vi "Target Vision Processing.vi"(3 "Particle Measurements (COG)":dbl[][](array[numeric]) format="%.2f", 5 "Rectangles (Shape Detection 1)":T1(array[cluster]) {"Corners"."Y" format="%.2f"; "Corners"."X" format="%.2f"}) -> (0 "Chosen X":dbl, 1 "Chosen Distance":dbl, 2 "High Y":dbl)   [LabVIEW 2012]
panel:
  in  "Numeric":dbl
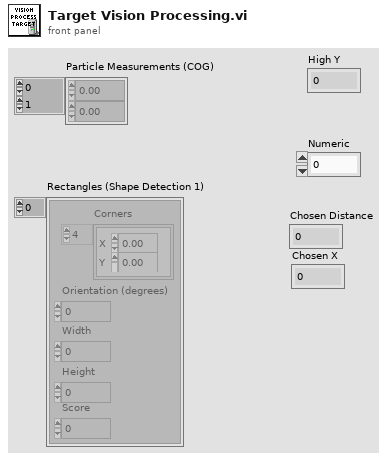
[diagram p1: front panel]
types:
  T1 = cluster{"Corners":cluster{"X":sgl, "Y":sgl}[], "Orientation (degrees)":dbl, "Width":dbl, "Height":dbl, "Score":dbl}[]
  T2 = cluster{"Rectangles (Shape Detection 1)[0]":cluster{"Corners":cluster{"X":sgl, "Y":sgl}[], "Orientation (degrees)":dbl, "Width":dbl, "Height":dbl, "Score":dbl}, "Rectangles (Shape Detection 1)[1]":cluster{"Corners":cluster{"X":sgl, "Y":sgl}[], "Orientation (degrees)":dbl, "Width":dbl, "Height":dbl, "Score":dbl}, "Rectangles (Shape Detection 1)[2]":cluster{"Corners":cluster{"X":sgl, "Y":sgl}[], "Orientation (degrees)":dbl, "Width":dbl, "Height":dbl, "Score":dbl}, "Rectangles (Shape Detection 1)[3]":cluster{"Corners":cluster{"X":sgl, "Y":sgl}[], "Orientation (degrees)":dbl, "Width":dbl, "Height":dbl, "Score":dbl}, "Rectangles (Shape Detection 1)[4]":cluster{"Corners":cluster{"X":sgl, "Y":sgl}[], "Orientation (degrees)":dbl, "Width":dbl, "Height":dbl, "Score":dbl}, "Rectangles (Shape Detection 1)[5]":cluster{"Corners":cluster{"X":sgl, "Y":sgl}[], "Orientation (degrees)":dbl, "Width":dbl, "Height":dbl, "Score":dbl}, "Rectangles (Shape Detection 1)[6]":cluster{"Corners":cluster{"X":sgl, "Y":sgl}[], "Orientation (degrees)":dbl, "Width":dbl, "Height":dbl, "Score":dbl}, "Rectangles (Shape Detection 1)[7]":cluster{"Corners":cluster{"X":sgl, "Y":sgl}[], "Orientation (degrees)":dbl, "Width":dbl, "Height":dbl, "Score":dbl}, "Rectangles (Shape Detection 1)[8]":cluster{"Corners":cluster{"X":sgl, "Y":sgl}[], "Orientation (degrees)":dbl, "Width":dbl, "Height":dbl, "Score":dbl}}
  T3 = cluster{"Corners":cluster{"X":sgl, "Y":sgl}[], "Orientation (degrees)":dbl, "Width":dbl, "Height":dbl, "Score":dbl}
  T4 = cluster{"Corners[0]":cluster{"X":sgl, "Y":sgl}, "Corners[1]":cluster{"X":sgl, "Y":sgl}, "Corners[2]":cluster{"X":sgl, "Y":sgl}, "Corners[3]":cluster{"X":sgl, "Y":sgl}, "Corners[4]":cluster{"X":sgl, "Y":sgl}, "Corners[5]":cluster{"X":sgl, "Y":sgl}, "Corners[6]":cluster{"X":sgl, "Y":sgl}, "Corners[7]":cluster{"X":sgl, "Y":sgl}, "Corners[8]":cluster{"X":sgl, "Y":sgl}}
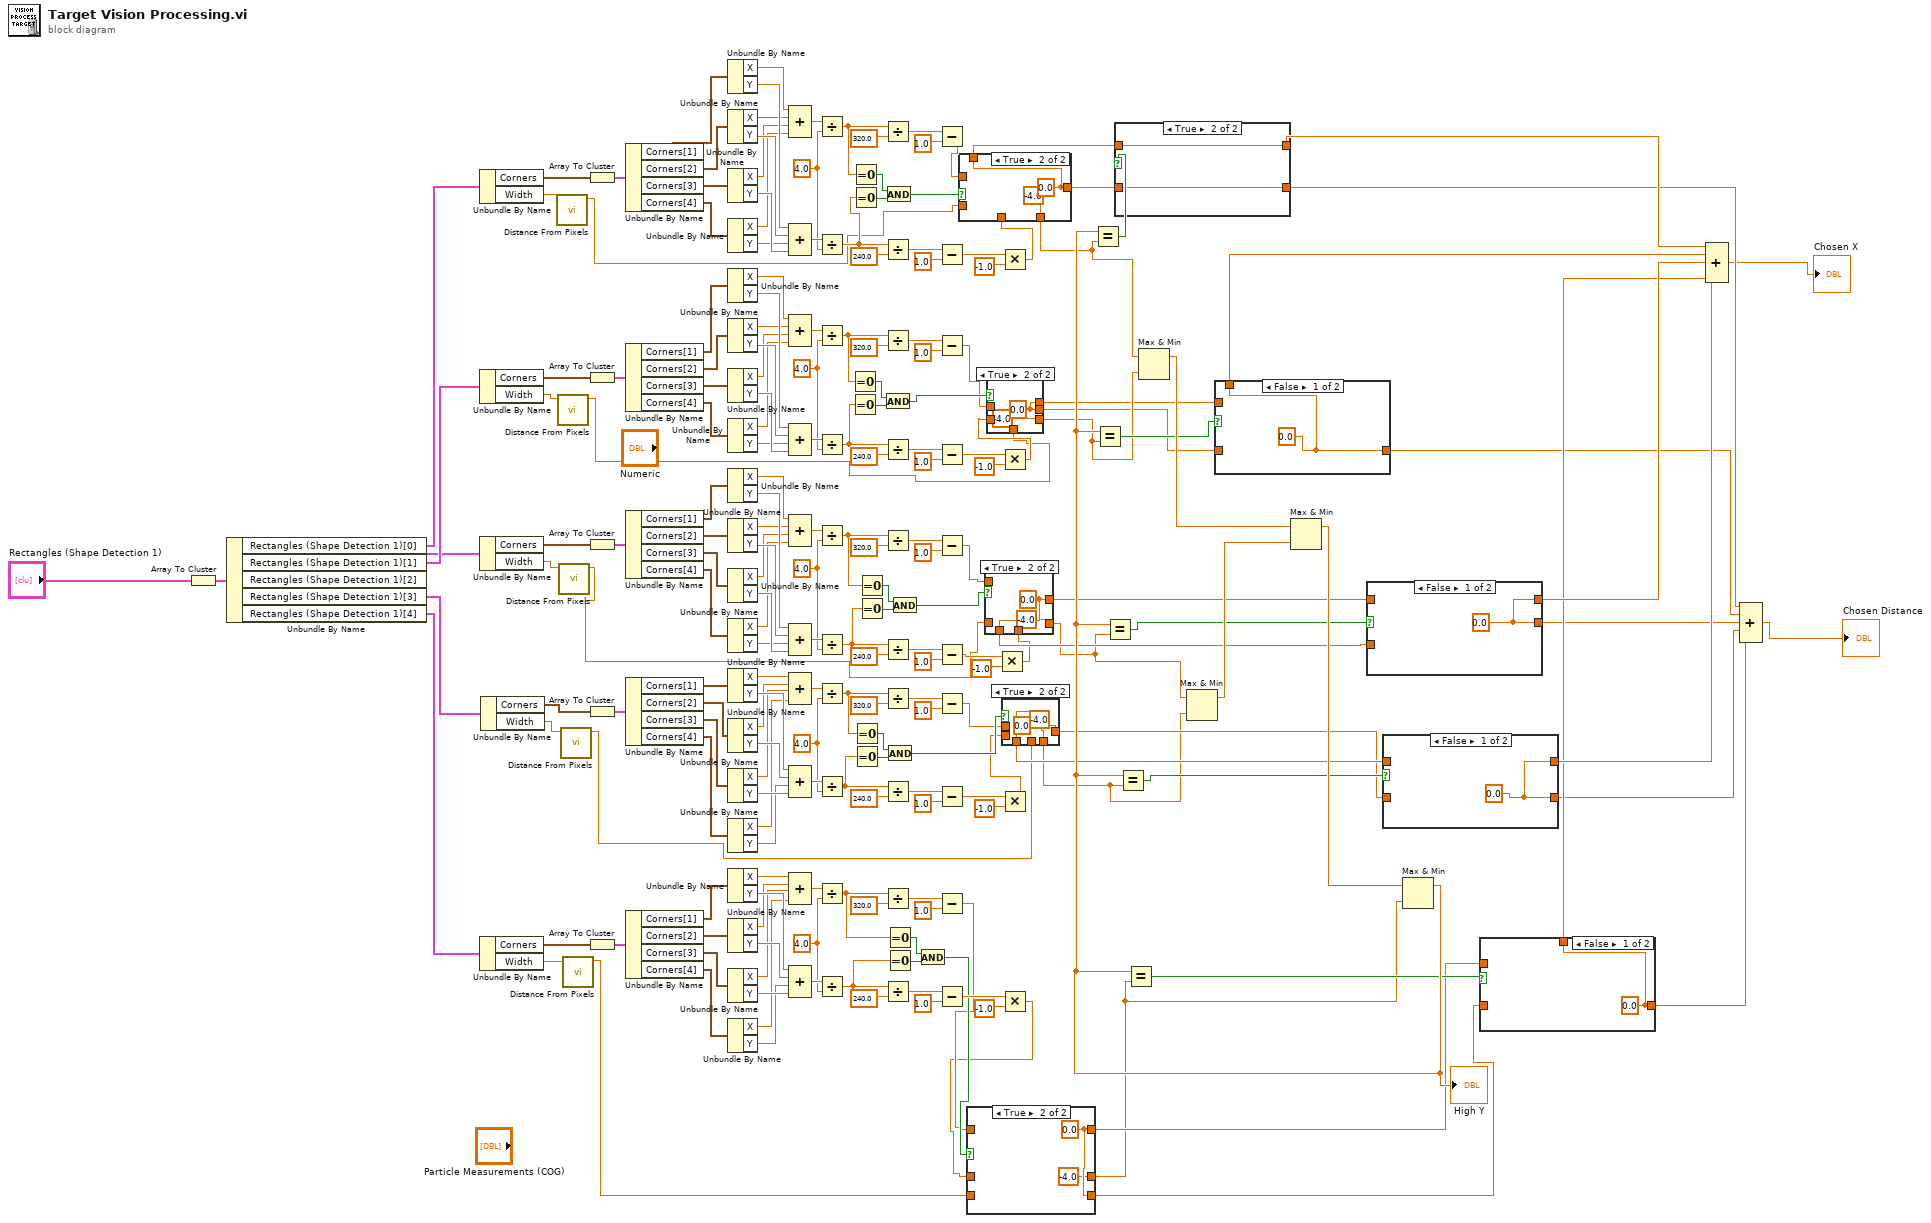
[diagram p0: block diagram]
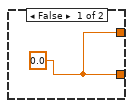
[diagram p11: hidden frame]
diagram:
  w92 = sgl 4.0 ("y")
  w117 = sgl 4.0 ("y")
  w141 = sgl 4.0 ("y")
  w166 = sgl 4.0 ("y")
  w190 = sgl 4.0 ("y")
  n1 = Array To Cluster(array="Rectangles (Shape Detection 1)") -> (cluster=w212:T2)
  n2 = Unbundle By Name(w212) -> ("Rectangles (Shape Detection 1)[0]"=w211:T3, "Rectangles (Shape Detection 1)[1]"=w210:T3, "Rectangles (Shape Detection 1)[2]"=w209:T3, "Rectangles (Shape Detection 1)[3]"=w208:T3, "Rectangles (Shape Detection 1)[4]"=w207:T3)
  n3 = Unbundle By Name(w211) -> ("Corners"=w206:cluster{"X":sgl, "Y":sgl}[], "Width"=w81:dbl)
  n4 = Unbundle By Name(w210) -> ("Corners"=w157:cluster{"X":sgl, "Y":sgl}[], "Width"=w77:dbl)
  n5 = Unbundle By Name(w209) -> ("Corners"=w133:cluster{"X":sgl, "Y":sgl}[], "Width"=w78:dbl)
  n6 = Unbundle By Name(w207) -> ("Corners"=w83:cluster{"X":sgl, "Y":sgl}[], "Width"=w80:dbl)
  n7 = Unbundle By Name(w208) -> ("Corners"=w108:cluster{"X":sgl, "Y":sgl}[], "Width"=w79:dbl)
  n8 = call "Distance From Pixels.vi"("Width"=w81) -> ("Distance"=w50:dbl)  [unwired: 10 in]
  n9 = call "Distance From Pixels.vi"("Width"=w77) -> ("Distance"=w23:dbl)  [unwired: 10 in]
  n10 = call "Distance From Pixels.vi"("Width"=w78) -> ("Distance"=w20:dbl)  [unwired: 10 in]
  n11 = call "Distance From Pixels.vi"("Width"=w79) -> ("Distance"=w11:dbl)  [unwired: 10 in]
  n12 = call "Distance From Pixels.vi"("Width"=w80) -> ("Distance"=w2:dbl)  [unwired: 10 in]
  n13 = Array To Cluster(array=w206) -> (cluster=w205:T4)
  n14 = Array To Cluster(array=w157) -> (cluster=w181:T4)
  n15 = Array To Cluster(array=w133) -> (cluster=w156:T4)
  n16 = Array To Cluster(array=w108) -> (cluster=w132:T4)
  n17 = Array To Cluster(array=w83) -> (cluster=w107:T4)
  n18 = Unbundle By Name(w205) -> ("Corners[1]"=w204:cluster{"X":sgl, "Y":sgl}, "Corners[2]"=w203:cluster{"X":sgl, "Y":sgl}, "Corners[3]"=w202:cluster{"X":sgl, "Y":sgl}, "Corners[4]"=w201:cluster{"X":sgl, "Y":sgl})
  n19 = Unbundle By Name(w181) -> ("Corners[1]"=w180:cluster{"X":sgl, "Y":sgl}, "Corners[2]"=w179:cluster{"X":sgl, "Y":sgl}, "Corners[3]"=w178:cluster{"X":sgl, "Y":sgl}, "Corners[4]"=w177:cluster{"X":sgl, "Y":sgl})
  n20 = Unbundle By Name(w156) -> ("Corners[1]"=w155:cluster{"X":sgl, "Y":sgl}, "Corners[2]"=w154:cluster{"X":sgl, "Y":sgl}, "Corners[3]"=w153:cluster{"X":sgl, "Y":sgl}, "Corners[4]"=w152:cluster{"X":sgl, "Y":sgl})
  n21 = Unbundle By Name(w132) -> ("Corners[1]"=w131:cluster{"X":sgl, "Y":sgl}, "Corners[2]"=w130:cluster{"X":sgl, "Y":sgl}, "Corners[3]"=w129:cluster{"X":sgl, "Y":sgl}, "Corners[4]"=w128:cluster{"X":sgl, "Y":sgl})
  n22 = Unbundle By Name(w107) -> ("Corners[1]"=w106:cluster{"X":sgl, "Y":sgl}, "Corners[2]"=w105:cluster{"X":sgl, "Y":sgl}, "Corners[3]"=w104:cluster{"X":sgl, "Y":sgl}, "Corners[4]"=w103:cluster{"X":sgl, "Y":sgl})
  n23 = Unbundle By Name(w204) -> ("X"=w200:sgl, "Y"=w199:sgl)
  n24 = Unbundle By Name(w203) -> ("X"=w198:sgl, "Y"=w197:sgl)
  n25 = Unbundle By Name(w202) -> ("X"=w196:sgl, "Y"=w195:sgl)
  n26 = Unbundle By Name(w201) -> ("X"=w194:sgl, "Y"=w193:sgl)
  n27 = Unbundle By Name(w180) -> ("X"=w176:sgl, "Y"=w175:sgl)
  n28 = Unbundle By Name(w179) -> ("X"=w174:sgl, "Y"=w173:sgl)
  n29 = Unbundle By Name(w178) -> ("X"=w172:sgl, "Y"=w171:sgl)
  n30 = Unbundle By Name(w177) -> ("X"=w170:sgl, "Y"=w169:sgl)
  n31 = Unbundle By Name(w155) -> ("X"=w151:sgl, "Y"=w150:sgl)
  n32 = Unbundle By Name(w154) -> ("X"=w149:sgl, "Y"=w148:sgl)
  n33 = Unbundle By Name(w153) -> ("X"=w147:sgl, "Y"=w146:sgl)
  n34 = Unbundle By Name(w152) -> ("X"=w145:sgl, "Y"=w144:sgl)
  n35 = Unbundle By Name(w131) -> ("X"=w127:sgl, "Y"=w126:sgl)
  n36 = Unbundle By Name(w130) -> ("X"=w125:sgl, "Y"=w124:sgl)
  n37 = Unbundle By Name(w129) -> ("X"=w123:sgl, "Y"=w122:sgl)
  n38 = Unbundle By Name(w128) -> ("X"=w121:sgl, "Y"=w120:sgl)
  n39 = Unbundle By Name(w106) -> ("X"=w102:sgl, "Y"=w101:sgl)
  n40 = Unbundle By Name(w105) -> ("X"=w100:sgl, "Y"=w99:sgl)
  n41 = Unbundle By Name(w104) -> ("X"=w98:sgl, "Y"=w97:sgl)
  n42 = Unbundle By Name(w103) -> ("X"=w96:sgl, "Y"=w95:sgl)
  n43 = Compound Arithmetic op=ADD(w200, w198, w196, w194) -> (w192:sgl)
  n44 = Compound Arithmetic op=ADD(w199, w197, w193, w195) -> (w191:sgl)
  n45 = Compound Arithmetic op=ADD(w176, w174, w172, w170) -> (w168:sgl)
  n46 = Compound Arithmetic op=ADD(w175, w173, w169, w171) -> (w167:sgl)
  n47 = Compound Arithmetic op=ADD(w151, w149, w147, w145) -> (w143:sgl)
  n48 = Compound Arithmetic op=ADD(w150, w148, w144, w146) -> (w142:sgl)
  n49 = Compound Arithmetic op=ADD(w127, w125, w123, w121) -> (w119:sgl)
  n50 = Compound Arithmetic op=ADD(w126, w124, w120, w122) -> (w118:sgl)
  n51 = Compound Arithmetic op=ADD(w102, w100, w98, w96) -> (w94:sgl)
  n52 = Compound Arithmetic op=ADD(w101, w99, w95, w97) -> (w93:sgl)
  n53 = Divide(x=w192, y=w190) -> (x/y=w52:sgl)
  n54 = Divide(x=w191, y=w190) -> (x/y=w51:sgl)
  n55 = Divide(x=w168, y=w166) -> (x/y=w30:sgl)
  n56 = Divide(x=w167, y=w166) -> (x/y=w29:sgl)
  n57 = Divide(x=w143, y=w141) -> (x/y=w32:sgl)
  n58 = Divide(x=w142, y=w141) -> (x/y=w31:sgl)
  n59 = Divide(x=w119, y=w117) -> (x/y=w34:sgl)
  n60 = Divide(x=w118, y=w117) -> (x/y=w33:sgl)
  n61 = Divide(x=w94, y=w92) -> (x/y=w36:sgl)
  n62 = Divide(x=w93, y=w92) -> (x/y=w35:sgl)
  n63 = Equal To 0?(x=w30) -> (x = 0?=w44:bool)
  n64 = Equal To 0?(x=w29) -> (x = 0?=w43:bool)
  n65 = Equal To 0?(x=w52) -> (x = 0?=w55:bool)
  n66 = Equal To 0?(x=w51) -> (x = 0?=w54:bool)
  n67 = Equal To 0?(x=w34) -> (x = 0?=w40:bool)
  n68 = Equal To 0?(x=w33) -> (x = 0?=w39:bool)
  n69 = Equal To 0?(x=w32) -> (x = 0?=w42:bool)
  n70 = Equal To 0?(x=w31) -> (x = 0?=w41:bool)
  n71 = Divide(x=w52, y=sgl 320.0) -> (x/y=w188:sgl)
  n72 = Divide(x=w51, y=sgl 240.0) -> (x/y=w185:sgl)
  n73 = Divide(x=w30, y=sgl 320.0) -> (x/y=w164:sgl)
  n74 = And(x=w44, y=w43) -> (x .and. y?=w28:bool)
  n75 = Divide(x=w29, y=sgl 240.0) -> (x/y=w161:sgl)
  n76 = Divide(x=w32, y=sgl 320.0) -> (x/y=w139:sgl)
  n77 = Divide(x=w31, y=sgl 240.0) -> (x/y=w136:sgl)
  n78 = Divide(x=w34, y=sgl 320.0) -> (x/y=w115:sgl)
  n79 = Divide(x=w33, y=sgl 240.0) -> (x/y=w112:sgl)
  n80 = Divide(x=w36, y=sgl 320.0) -> (x/y=w90:sgl)
  n81 = Divide(x=w35, y=sgl 240.0) -> (x/y=w87:sgl)
  n82 = And(x=w55, y=w54) -> (x .and. y?=w53:bool)
  n83 = And(x=w40, y=w39) -> (x .and. y?=w14:bool)
  n84 = Equal To 0?(x=w36) -> (x = 0?=w38:bool)
  n85 = Equal To 0?(x=w35) -> (x = 0?=w37:bool)
  n86 = And(x=w42, y=w41) -> (x .and. y?=w21:bool)
  n87 = And(x=w38, y=w37) -> (x .and. y?=w7:bool)
  n88 = Subtract(x=w188, y=sgl 1.0) -> (x-y=w48:sgl)
  n89 = Subtract(x=w185, y=sgl 1.0) -> (x-y=w183:sgl)
  n90 = Subtract(x=w164, y=sgl 1.0) -> (x-y=w25:sgl)
  n91 = Subtract(x=w161, y=sgl 1.0) -> (x-y=w159:sgl)
  n92 = Subtract(x=w139, y=sgl 1.0) -> (x-y=w18:sgl)
  n93 = Subtract(x=w136, y=sgl 1.0) -> (x-y=w82:sgl)
  n94 = Subtract(x=w115, y=sgl 1.0) -> (x-y=w13:sgl)
  n95 = Subtract(x=w112, y=sgl 1.0) -> (x-y=w110:sgl)
  n96 = Subtract(x=w90, y=sgl 1.0) -> (x-y=w6:sgl)
  n97 = Subtract(x=w87, y=sgl 1.0) -> (x-y=w85:sgl)
  n98 = Multiply(x=w82, y=sgl -1.0) -> (x*y=w16:sgl)
  n99 = case shown="True" w21 {
    tunnel: w20 -> [w216 _]
    tunnel: [w216 w218] -> w19
    tunnel: w18 -> [w215 _]
    tunnel: [w215 w218] -> w17
    tunnel: w16 -> [w214 _]
    tunnel: [w214 sgl -4.0] -> w15
    frame False {
    }
    frame True {
      w218 = sgl 0.0
    }
  }
  n100 = Multiply(x=w183, y=sgl -1.0) -> (x*y=w49:sgl)
  n101 = case shown="True" w53 {
    tunnel: w50 -> [w220 _]
    tunnel: w49 -> [w219 _]
    tunnel: w48 -> [w221 _]
    tunnel: [w221 w223] -> w47
    tunnel: [w220 w223] -> w46
    tunnel: [w219 sgl -4.0] -> w45
    frame False {
    }
    frame True {
      w223 = 0.0 ("Distance")
    }
  }
  n102 = Multiply(x=w159, y=sgl -1.0) -> (x*y=w27:sgl)
  n103 = case shown="True" w28 {
    tunnel: w27 -> [w226 _]
    tunnel: [w226 sgl -4.0] -> w26
    tunnel: w25 -> [w225 _]
    tunnel: [w225 w228] -> w24
    tunnel: w23 -> [w224 _]
    tunnel: [w224 w228] -> w22
    frame False {
    }
    frame True {
      w228 = 0.0 ("Distance")
    }
  }
  n104 = Multiply(x=w110, y=sgl -1.0) -> (x*y=w9:sgl)
  n105 = Multiply(x=w85, y=sgl -1.0) -> (x*y=w4:sgl)
  n106 = case shown="True" w7 {
    tunnel: w6 -> [w231 _]
    tunnel: [w231 w233] -> w5
    tunnel: w4 -> [w230 _]
    tunnel: [w230 sgl -4.0] -> w3
    tunnel: w2 -> [w229 _]
    tunnel: [w229 w233] -> w1
    frame False {
    }
    frame True {
      w233 = sgl 0.0
    }
  }
  n107 = case shown="True" w14 {
    tunnel: w13 -> [w236 _]
    tunnel: [w236 w238] -> w12
    tunnel: w11 -> [w235 _]
    tunnel: [w235 w238] -> w10
    tunnel: w9 -> [w234 _]
    tunnel: [w234 sgl -4.0] -> w8
    frame False {
    }
    frame True {
      w238 = 0.0 ("Distance")
    }
  }
  n108 = Max & Min(x=w45, y=w26) -> (max(x,y)=w76:sgl)  [unwired: 1 out]
  n109 = Max & Min(x=w15, y=w8) -> (max(x,y)=w75:sgl)  [unwired: 1 out]
  n110 = Max & Min(x=w76, y=w75) -> (max(x,y)=w74:sgl)  [unwired: 1 out]
  n111 = Max & Min(x=w74, y=w3) -> (max(x,y)=w73:sgl)  [unwired: 1 out]
  "High Y" <- w73
  n112 = Equal?(x=w73, y=w45) -> (x = y?=w72:bool)
  n113 = Equal?(x=w73, y=w26) -> (x = y?=w71:bool)
  n114 = Equal?(x=w73, y=w15) -> (x = y?=w70:bool)
  n115 = case shown="True" w72 {
    tunnel: w47 -> [_ w241]
    tunnel: w46 -> [_ w240]
    tunnel: [w239 w241] -> w67
    tunnel: [w239 w240] -> w62
    frame False {
      w239 = 0.0 ("Distance")
    }
    frame True {
    }
  }
  n116 = Equal?(x=w73, y=w8) -> (x = y?=w69:bool)
  n117 = Equal?(x=w73, y=w3) -> (x = y?=w68:bool)
  n118 = case shown="False" w71 {
    tunnel: w24 -> [_ w244]
    tunnel: w22 -> [_ w243]
    tunnel: [w242 w244] -> w66
    tunnel: [w242 w243] -> w61
    frame False {
      w242 = 0.0 ("Distance")
    }
    frame True {
    }
  }
  n119 = case shown="False" w70 {
    tunnel: w17 -> [_ w247]
    tunnel: w19 -> [_ w246]
    tunnel: [w245 w247] -> w65
    tunnel: [w245 w246] -> w60
    frame False {
      w245 = 0.0 ("Distance")
    }
    frame True {
    }
  }
  n120 = case shown="False" w69 {
    tunnel: w12 -> [_ w250]
    tunnel: w10 -> [_ w249]
    tunnel: [w248 w250] -> w64
    tunnel: [w248 w249] -> w59
    frame False {
      w248 = 0.0 ("Distance")
    }
    frame True {
    }
  }
  n121 = case shown="False" w68 {
    tunnel: w5 -> [_ w253]
    tunnel: w1 -> [_ w252]
    tunnel: [w251 w253] -> w63
    tunnel: [w251 w252] -> w58
    frame False {
      w251 = 0.0 ("Distance")
    }
    frame True {
    }
  }
  n122 = Compound Arithmetic op=ADD(w67, w66, w65, w64, w63) -> (→"Chosen X":dbl)
  n123 = Compound Arithmetic op=ADD(w62, w61, w60, w59, w58) -> (→"Chosen Distance":dbl)
